vi "PIM Print Panel.vi"(7 "VI Panel Ref":refnum<vi>, 9 "DisplayMode":T1 items=["Spectral", "Strip Chart", "Swept Frequency"], 10 "IM Plot Ref":refnum<vi>, 11 "Peak Slider Ref":refnum<vi>) -> ()   [LabVIEW 2011]
uses:
  BPIMCore/Display/PIM Display Mode.ctl
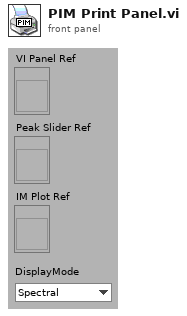
[diagram p1: front panel]
types:
  T1 = typedef "PIM Display Mode.ctl" = u16
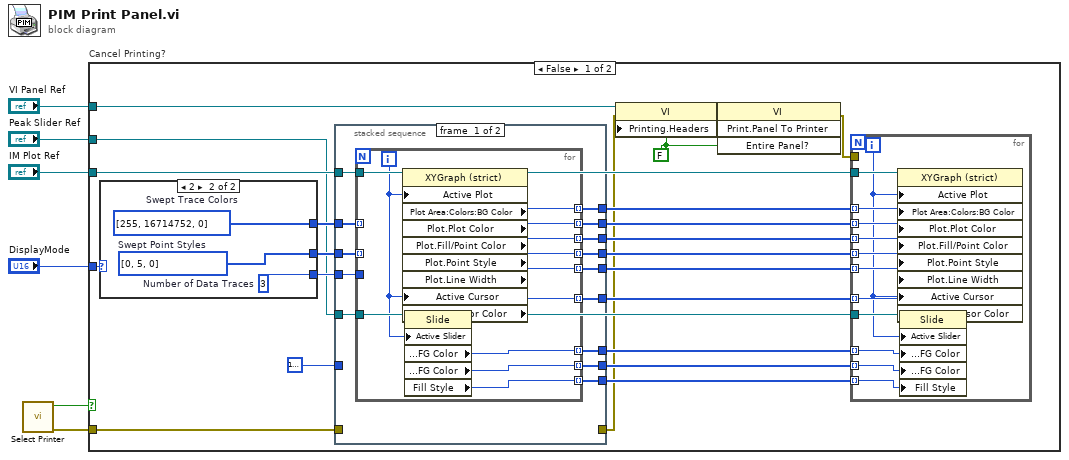
[diagram p0: block diagram]
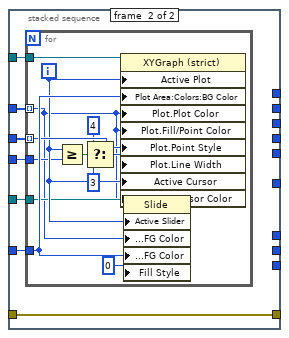
[diagram p2: hidden frame]
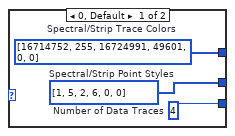
[diagram p3: hidden frame]
diagram:
  n1 = call "Select Printer.vi"() -> ("error out"=w1:errorcluster, "Canceled?"=w2:bool)  [unwired: 1 in, 9 out]
  n2 = case "Cancel Printing?" shown="False" w2 {
    tunnel: "DisplayMode" -> [w23 _]
    tunnel: "VI Panel Ref" -> [w7 _]
    tunnel: "IM Plot Ref" -> [w22 _]
    tunnel: "Peak Slider Ref" -> [w21 _]
    tunnel: w1 -> [w9 _]
    frame False {
      w24 = FALSE ("Entire Panel?")
      n3 = case shown="2" w23 {
        tunnel: [w89 w91] -> w26
        tunnel: [w88 w90] -> w28
        tunnel: [w87 w92] -> w29
        frame 0, Default {
          w87 = 4  # Number of Data Traces
          w88 = u8[] [1, 5, 2, 6, 0, 0]  # Spectral/Strip Point Styles
          w89 = u32[] [16714752, 255, 16724991, 49601, 0, 0]  # Spectral/Strip Trace Colors
        }
        frame 2 {
          w90 = u8[] [0, 5, 0]  # Swept Point Styles
          w91 = u32[] [255, 16714752, 0]  # Swept Trace Colors
          w92 = 3  # Number of Data Traces
        }
      }
      n4 = stacked-sequence {
        tunnel: w29 -> [w53 w74]
        tunnel: w28 -> [w54 w73]
        tunnel: u32 16777226 -> [_ w72]
        tunnel: w26 -> [w55 w71]
        tunnel: w22 -> [w51 w70]
        tunnel: w21 -> [w52 w69]
        tunnel: [w50 _] -> w20
        tunnel: [w49 _] -> w19
        tunnel: [w48 _] -> w18
        tunnel: [w47 _] -> w17
        tunnel: [w46 _] -> w16
        tunnel: [w45 _] -> w15
        tunnel: [w44 _] -> w14
        tunnel: [w43 _] -> w13
        tunnel: [w42 _] -> w12
        tunnel: w9 -> [_ w68]
        tunnel: [_ w68] -> w8
        frame #0 {
          n5 = for {
            tunnel: w55 -> [_] mode=indexing
            tunnel: w54 -> [_] mode=indexing
            tunnel: w53 -> [_]
            tunnel: w52 -> [w67]
            tunnel: w51 -> [w66]
            tunnel: [w65] -> w50 mode=indexing
            tunnel: [w64] -> w49 mode=indexing
            tunnel: [w63] -> w48 mode=indexing
            tunnel: [w62] -> w47 mode=indexing
            tunnel: [w61] -> w46 mode=indexing
            tunnel: [w60] -> w45 mode=indexing
            tunnel: [w59] -> w44 mode=indexing
            tunnel: [w58] -> w43 mode=indexing
            tunnel: [w57] -> w42 mode=indexing
            i -> [w56]
            n6 = property on="Property Node" class="XYGraph (strict)"(reference=w66, "Active Plot"=w56, "Active Cursor"=w56) -> ("Plot Area:Colors:BG Color"=w65:u32, "Plot.Plot Color"=w64:u32, "Plot.Fill/Point Color"=w63:u32, "Plot.Point Style"=w62:u8, "Plot.Line Width"=w61:u8, "Cursor.Cursor Color"=w60:u32)  [unwired: 1 in, 2 out]
            n7 = property on="Property Node" class="Slide"(reference=w67, "Active Slider"=w56) -> ("Slider Colors:FG Color"=w59:u32, "Housing Colors:FG Color"=w58:u32, "Fill Style"=w57:i32)  [unwired: 1 in, 2 out]
          }
        }
        frame #1 {
          n8 = for {
            tunnel: w72 -> [w85]
            tunnel: w71 -> [w75] mode=indexing
            tunnel: w73 -> [w84] mode=indexing
            tunnel: w74 -> [w82]
            tunnel: w70 -> [w77]
            tunnel: w69 -> [w76]
            i -> [w83]
            n9 = Greater Or Equal?(x=w83, y=w82) -> (x >= y?=w81:bool)
            n10 = Select(t=4 ("Fill Style"), s=w81, f=3 ("Fill Style")) -> (s? t:f=w78:i32)
            n11 = property on="Property Node" class="XYGraph (strict)"(reference=w77, "Active Plot"=w83, "Plot Area:Colors:BG Color"=w85, "Plot.Plot Color"=w75, "Plot.Fill/Point Color"=w75, "Plot.Point Style"=w84, "Plot.Line Width"=w78, "Active Cursor"=w83, "Cursor.Cursor Color"=w75) -> ()  [unwired: 1 in, 2 out]
            n12 = property on="Property Node" class="Slide"(reference=w76, "Active Slider"=w83, "Slider Colors:FG Color"=w75, "Housing Colors:FG Color"=w85, "Fill Style"=0) -> ()  [unwired: 1 in, 2 out]
          }
        }
      }
      n13 = property class="VI"(reference=w7, error in=w8, "Printing.Headers"=w24) -> (reference out=w10:refnum<vi>, error out=w25:errorcluster)
      n14 = invoke class="VI" method="Print.Panel To Printer"(reference=w10, error in=w25, "Entire Panel?"=w24) -> (error out=w11:errorcluster)  [unwired: 1 in, 3 out]
      n15 = for {
        tunnel: w21 -> [w41]
        tunnel: w22 -> [w40]
        tunnel: w20 -> [w39] mode=indexing
        tunnel: w19 -> [w38] mode=indexing
        tunnel: w18 -> [w37] mode=indexing
        tunnel: w17 -> [w36] mode=indexing
        tunnel: w16 -> [w35] mode=indexing
        tunnel: w15 -> [w34] mode=indexing
        tunnel: w14 -> [w33] mode=indexing
        tunnel: w13 -> [w32] mode=indexing
        tunnel: w12 -> [w31] mode=indexing
        tunnel: w11 -> [_]
        i -> [w30]
        n16 = property on="Property Node" class="XYGraph (strict)"(reference=w40, "Active Plot"=w30, "Plot Area:Colors:BG Color"=w39, "Plot.Plot Color"=w38, "Plot.Fill/Point Color"=w37, "Plot.Point Style"=w36, "Plot.Line Width"=w35, "Active Cursor"=w30, "Cursor.Cursor Color"=w34) -> ()  [unwired: 1 in, 2 out]
        n17 = property on="Property Node" class="Slide"(reference=w41, "Active Slider"=w30, "Slider Colors:FG Color"=w33, "Housing Colors:FG Color"=w32, "Fill Style"=w31) -> ()  [unwired: 1 in, 2 out]
      }
    }
    frame True {
    }
  }
